vi "Read Position.vi"(8 "error in (no error)":errorcluster, 11 "Grove 6 Axis Gyro Accel LSM6DS3 in":refnum<class "Grove 6 Axis Gyro Accel LSM6DS3.lvclass">) -> (0 "error out":errorcluster, 2 "Array":dbl[](array[numeric]) format="%.2f", 3 "Grove 6 Axis Gyro Accel LSM6DS3 out":refnum<class "Grove 6 Axis Gyro Accel LSM6DS3.lvclass">)   [LabVIEW 2020, in "CTI-Peripheral.lvlib" / "Grove 6 Axis Gyro Accel LSM6DS3.lvclass"]
uses:
  Grove 6 Axis Gyro Accel LSM6DS3.lvclass
  Grove 6 Axis Gyro Accel LSM6DS3.lvclass/Grove 6 Axis Gyro Accel LSM6DS3.ctl
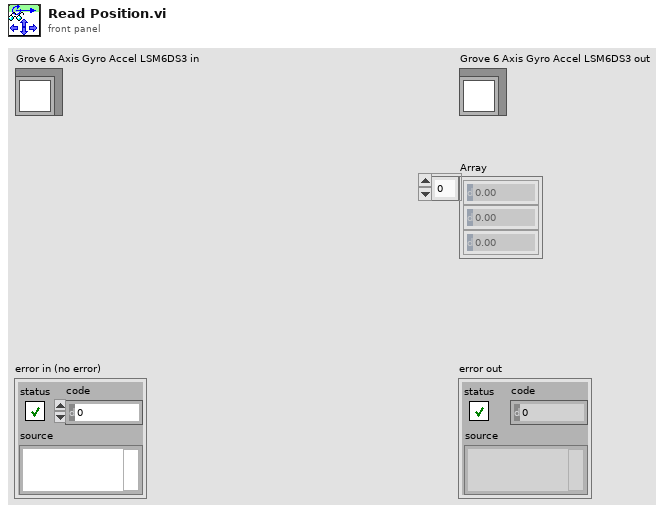
[diagram p1: front panel]
types:
  T1 = enum16{"No Register - Error", "D6D_SRC", "STATUS_REG", "OUT_TEMP_L", "OUT_TEMP_H", "OUTX_L_G", "OUTX_H_G", "OUTY_L_G", "OUTY_H_G", "OUTZ_L_G", "OUTZ_H_G", "OUTX_L_XL", "OUTX_H_XL", "OUTY_L_XL", "OUTY_H_XL", "OUTZ_L_XL", "OUTZ_H_XL", "SENSORHUB1_REG", "SENSORHUB2_REG", "SENSORHUB3_REG", "SENSORHUB4_REG", "SENSORHUB5_REG", "SENSORHUB6_REG", "SENSORHUB7_REG", "SENSORHUB8_REG", "SENSORHUB9_REG", "SENSORHUB10_REG", "SENSORHUB11_REG", "SENSORHUB12_REG"}[]
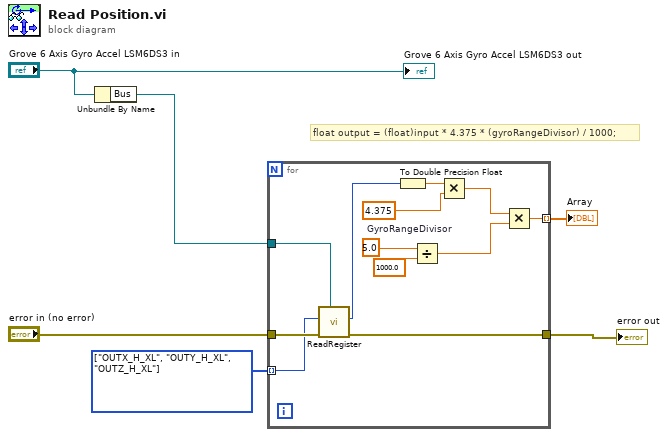
[diagram p0: block diagram]
diagram:
  w5 = T1 [enum."OUTX_H_XL", enum."OUTY_H_XL", enum."OUTZ_H_XL"] items=["No Register - Error", "D6D_SRC", "STATUS_REG", "OUT_TEMP_L", "OUT_TEMP_H", "OUTX_L_G", "OUTX_H_G", "OUTY_L_G", "OUTY_H_G", "OUTZ_L_G", "OUTZ_H_G", "OUTX_L_XL", "OUTX_H_XL", "OUTY_L_XL", "OUTY_H_XL", "OUTZ_L_XL", "OUTZ_H_XL", "SENSORHUB1_REG", "SENSORHUB2_REG", "SENSORHUB3_REG", "SENSORHUB4_REG", "SENSORHUB5_REG", "SENSORHUB6_REG", "SENSORHUB7_REG", "SENSORHUB8_REG", "SENSORHUB9_REG", "SENSORHUB10_REG", "SENSORHUB11_REG", "SENSORHUB12_REG"]
  # "float output = (float)input * 4.375 * (gyroRangeDivisor) / 1000;"
  n1 = Unbundle By Name("Grove 6 Axis Gyro Accel LSM6DS3 in") -> ("Bus"=w2:refnum<class "I2C Connection.lvclass">)
  n2 = for {
    tunnel: w5 -> [w8] mode=indexing
    tunnel: [w12] -> w4 mode=indexing
    tunnel: "error in (no error)" -> [w10]
    tunnel: [w11] -> w1
    tunnel: w2 -> [w9]
    w16 = 5.0  # GyroRangeDivisor
    n3 = call "ReadRegister.vi"("I2C Connection"=w9, "error in (no error)"=w10, "Register"=w8) -> ("error out"=w11:errorcluster, "Numeric"=w7:i16)  [unwired: 7 in]
    n4 = To Double Precision Float(number=w7) -> (double precision float=w18:dbl)
    n5 = Divide(x=w16, y=1000.0) -> (x/y=w14:dbl)
    n6 = Multiply(x=w18, y=4.375) -> (x*y=w13:dbl)
    n7 = Multiply(x=w13, y=w14) -> (x*y=w12:dbl)
  }
  "error out" <- w1
  "Array" <- w4
  "Grove 6 Axis Gyro Accel LSM6DS3 out" <- "Grove 6 Axis Gyro Accel LSM6DS3 in"
